vi "CPP_AeroFlow.vi"(5 "Pressure (mBar)":dbl=1000.0, 6 "Probe:Euler:Angles":T1, 7 "Temperature (C)":dbl=20.0, 9 "Calibration Folder Path":path=path "", 10 "Probe Type":T3=5 items=["5-Hole Probe"=5, "OmniProbe"=12], 11 "zeroedPress":dbl[][](array[numeric])=array820x5[4100 elements] caption="ZeroedPressures (mmH2O)") -> (0 "TotalPoints":i32, 1 "nGoodAF":i16, 2 "Output":T2, 4 "Time(ms)":u32)   [LabVIEW 2022 SP3]
doc: "Reduces pressure data to velocity components. There may be fewer reduced points than there were presures, due to failures in the reduction routine. This means the returned data should be NaN-clean, and ready for stats to be calculated. However take care if plotting velocities to the same timebase as pressures- gaps will have to be re-introduced"
uses:
  Controls/AeroprobeType.ctl
  eulerAngles.ctl
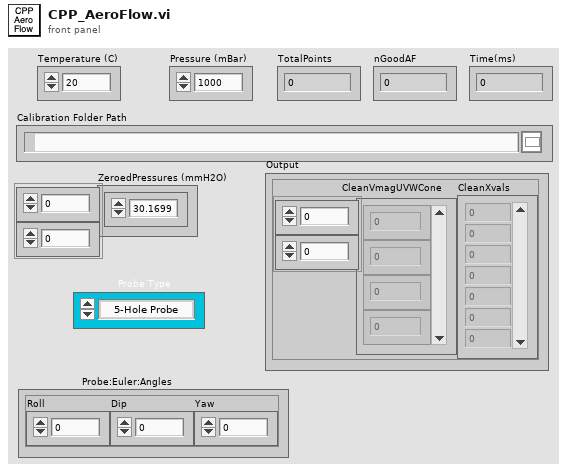
[diagram p1: front panel]
types:
  T1 = typedef "eulerAngles.ctl" = cluster{"Roll":dbl, "Dip":dbl, "Yaw":dbl}
  T2 = cluster{"CleanVmagUVWCone":dbl[][], "CleanXvals":i32[]}
  T3 = typedef "AeroprobeType.ctl" = u16
  T4 = cluster{"   Vmag          U               V              W        Cone":dbl[][], "Xvals":i32[]}
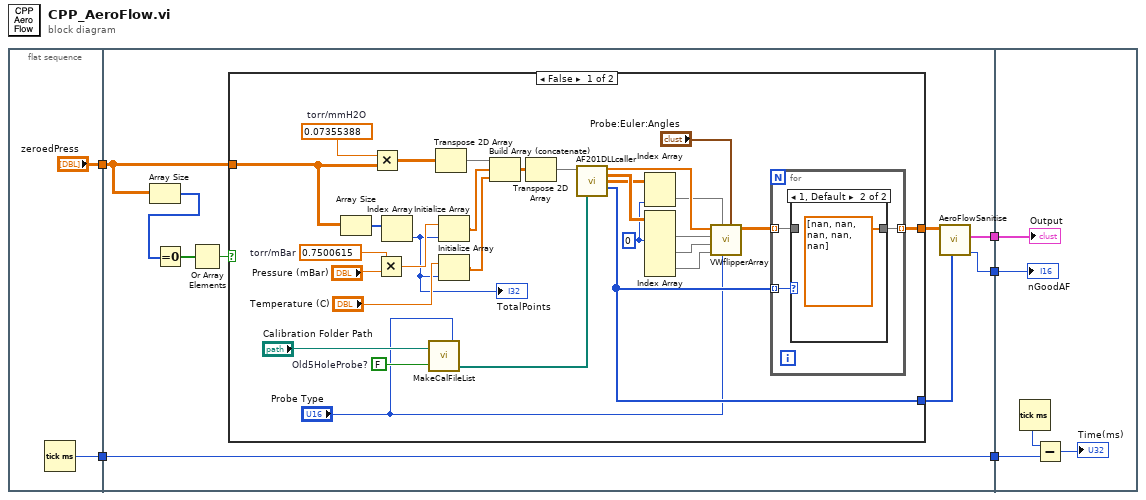
[diagram p0: block diagram]
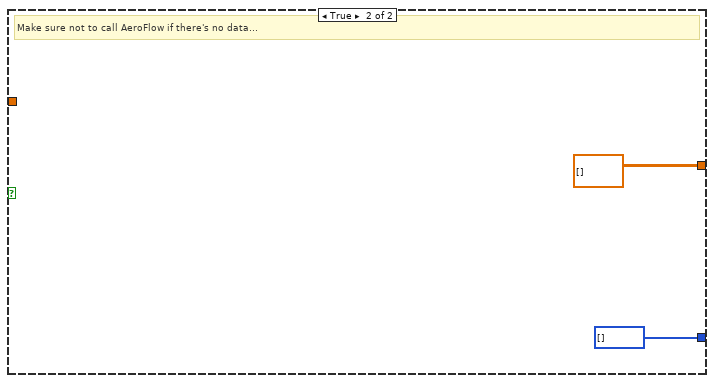
[diagram p3: hidden frame]
diagram:
  n1 = flat-sequence {
    tunnel: [w7] -> w5
    tunnel: ["zeroedPress"] -> w3
    tunnel: w5 -> [w11]
    tunnel: [w11] -> w4
    tunnel: w3 -> [w10]
    tunnel: [w9] -> w2
    tunnel: [w8] -> w1
    tunnel: w4 -> [w57]
    tunnel: w2 -> [w55]
    tunnel: w1 -> [w54]
    frame #0 {
      n2 = Tick Count (ms)() -> (millisecond timer value=w7:u32)
    }
    frame #1 {
      n3 = Array Size(array=w10) -> (size(s)=w15:i32[])
      n4 = Equal To 0?(x=w15) -> (x = 0?=w16:bool[])
      n5 = Or Array Elements(Boolean array=w16) -> (logical OR=w14:bool)
      n6 = case shown="False" w14 {
        tunnel: w10 -> [w32 _]
        tunnel: [w20 dbl[][] [] ("VmagUVWCone")] -> w13
        tunnel: [w19 i32[] [] ("ErrorReduced")] -> w12
        frame False {
          w22 = 0 ("disabled index (col)")
          w44 = 0.7500615  # torr/mBar
          w43 = FALSE  # Old5HoleProbe?
          w24 = 0.07355388  # torr/mmH2O
          n7 = Array Size(array=w32) -> (size(s)=w29:i32[])
          n8 = Multiply(x=w24, y=w32) -> (x*y=w30:dbl[][])
          n9 = Multiply(x=w44, y="Pressure (mBar)") -> (x*y=w46:dbl)
          n10 = Index Array(array=w29) -> (element=w33:i32)  [unwired: 1 in]
          "TotalPoints" <- w33
          n11 = call "MakeCalFileList.vi"("Calibration Folder Path"="Calibration Folder Path", "Old5HoleProbe?"=w43, "Probe Type"="Probe Type") -> ("AeroFlowCals"=w38:path[])  [unwired: 1 out]
          n12 = Transpose 2D Array(2D array=w30) -> (transposed array=w25:dbl[][])
          n13 = Initialize Array(w46, w33) -> (w27:dbl[])
          n14 = Initialize Array("Temperature (C)", w33) -> (w26:dbl[])
          n15 = Build Array (concatenate)(w25, w27, w26) -> (w28:dbl[][])
          n16 = Transpose 2D Array(2D array=w28) -> (transposed array=w31:dbl[][])
          n17 = call "AF201DLLcaller.vi"("Data to Reduce"=w31, "Calibration File(s)"=w38) -> ("Vel_Mag_calc"=w37:dbl[], "UVW_calc"=w39:dbl[][], "angles_calc(Cone/Roll/Alpha/Beta)"=w35:dbl[][], "ErrorReduced"=w19:i32[])  [unwired: 9 in, 1 out]
          n18 = Index Array(array=w35, index (col)=w22) -> (element=w36:dbl[])  [unwired: 1 in]
          n19 = Index Array(array=w39, index (col) #1=w22) -> (element #1=w40:dbl[], element #2=w41:dbl[], element #3=w42:dbl[])  [unwired: 5 in]
          n20 = call "VWflipperArray.vi"("Probe:Euler:Angles"="Probe:Euler:Angles", "Probe Type"="Probe Type", "Theta Degree"=w36, "Probe w m/s"=w42, "Probe v m/s"=w41, "Probe u  m/s"=w40, "VMagn m/s"=w37) -> ("VmagUVWCone"=w21:dbl[][])  [unwired: 4 in]
          n21 = for {
            tunnel: w21 -> [w47] mode=indexing
            tunnel: w19 -> [w49] mode=indexing
            tunnel: [w48] -> w20 mode=indexing
            n22 = case shown="1, Default" w49 {
              tunnel: [w50 dbl[] [nan, nan, nan, nan, nan] ("VmagUVWCone")] -> w48
              tunnel: w47 -> [w50 _]
              frame 0 {
              }
              frame 1, Default {
              }
            }
          }
        }
        frame True {
          # "Make sure not to call AeroFlow if there's no data..."
        }
      }
      n23 = call "AeroFlowSanitise.vi"("ReductionCode"=w12, "RawReducedData"=w13) -> ("nGoodAF"=w8:i16, "CleanOutput"=w9:T4)  [unwired: 8 in]
    }
    frame #2 {
      n24 = Tick Count (ms)() -> (millisecond timer value=w58:u32)
      n25 = Subtract(x=w58, y=w57) -> (x-y=→"Time(ms)":u32)
      "nGoodAF" <- w54
      "Output" <- w55
    }
  }
